vi "ShooterMech v2.vi"() -> ()   [LabVIEW 2015]
uses:
  <vilib>/Rock Robotics/WPI/Solenoid/WPI_SolenoidValue.ctl
  <vilib>/Rock Robotics/WPI/Solenoid/WPI_SolenoidSetEnum.vi
  Velocity Variable.vi
panel:
  out "Shtr":dbl
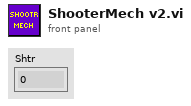
[diagram p1: front panel]
types:
  T1 = typedef "WPI_SolenoidValue.ctl" = enum16{"Off", "On", "Forward", "Reverse"}
  T2 = typedef "WPI_JoystickDevRef.ctl" = cluster{"Device":T3}
  T3 = typedef "WPI_JoystickDeviceEnum.ctl" = enum16{"USB 0", "USB 1", "USB 2", "USB 3", "USB 4", "USB 5"}
  T4 = cluster{"Buttons[0]":bool, "Buttons[1]":bool, "Buttons[2]":bool, "Buttons[3]":bool, "Buttons[4]":bool, "Buttons[5]":bool, "Buttons[6]":bool, "Buttons[7]":bool, "Buttons[8]":bool}
  T5 = typedef "WPI_SolenoidDevRef.ctl" = cluster{"DevStatus":errorcluster, "Pneumatics Control Module":u8, "Forward Solenoid Channel":T6, "Reverse Solenoid Channel":T6}
  T6 = typedef "WPI_SolenoidChannel.ctl" = enum8{"Solenoid 0", "Solenoid 1", "Solenoid 2", "Solenoid 3", "Solenoid 4", "Solenoid 5", "Solenoid 6", "Solenoid 7", "Invalid"}
  T7 = typedef "WPI_MotorControlDeviceRef.ctl" = cluster{"DeviceStatus":errorcluster, "Type":T8, "PWM":cluster{"PWM Channel":T9, "DeadBand":T10}, "CAN":cluster{"Device Number":u8, "Control Mode":T11, "Semaphore":T12, "Max Vout":dbl, "TalonSRX Control Mode":T13}, "Invert":bool}
  T8 = typedef "WPI_MotorControlType.ctl" = enum16{"PWM", "CAN", "CANTalonSRX"}
  T9 = typedef "FPGA_DIOPWMChannel.ctl" = enum8{"PWM 0", "PWM 1", "PWM 2", "PWM 3", "PWM 4", "PWM 5", "PWM 6", "PWM 7", "PWM 8", "PWM 9", "PWM MXP 0", "PWM MXP 1", "PWM MXP 2", "PWM MXP 3", "PWM MXP 4", "PWM MXP 5", "PWM MXP 6", "PWM MXP 7", "PWM MXP 8", "PWM MXP 9", "Invalid"}
  T10 = typedef "WPI_PWMDeadband.ctl" = cluster{"Name":string, "maxPositivePwm":i32, "minPositivePwm":i32, "centerPwm":i32, "maxNegativePwm":i32, "minNegativePwm":i32, "angularRange":u16}
  T11 = typedef "WPI_CANJaguar_ControlMode.ctl" = enum8{"Percent VBus", "Current", "Speed", "Position", "Voltage"}
  T12 = typedef "Semaphore RefNum" = refnum<k1>
  T13 = typedef "WPI_CANTalonSRX_APIControlMode.ctl" = enum8{"Percent VBus", "Speed", "Position", "Slave", "Unchanged / Invalid", "Voltage Compensation", "Current", "Motion Profile"}
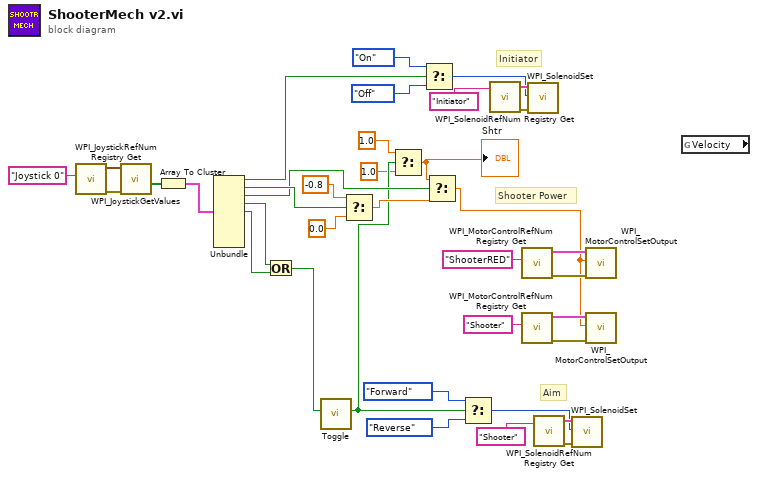
[diagram p0: block diagram]
diagram:
  # "Shooter Power"
  # "Aim"
  # "Initiator"
  n1 = call <vilib>:"WPI_JoystickRefNum Registry Get.vi"("refnum name"="Joystick 0") -> ("error out"=w25:errorcluster, "JoystickDevRef"=w24:T2)  [unwired: 9 in]
  n2 = call <vilib>:"WPI_JoystickGetValues.vi"("error in (no error)"=w25, "JoystickDevRef"=w24) -> ("Buttons"=w23:bool[])  [unwired: 5 in, 4 out]
  n3 = Array To Cluster(array=w23) -> (cluster=w22:T4)
  n4 = Unbundle(w22) -> ("Buttons[0]"=w10:bool, "Buttons[1]"=w9:bool, "Buttons[2]"=w8:bool, "Buttons[3]"=w6:bool, "Buttons[4]"=w7:bool)  [unwired: 4 out]
  n5 = Or(x=w6, y=w7) -> (x .or. y?=w5:bool)
  n6 = call "Toggle.vi"("Input"=w5) -> ("Output"=w3:bool)  [unwired: 10 in]
  n7 = Select(t=-0.8, s=w9, f=0.0) -> (s? t:f=w14:dbl)
  n8 = Select(t=1.0 ("Output"), s=w3, f=1.0) -> (s? t:f=w2:dbl)
  "Shtr" <- w2
  n9 = Select(t=WPI_SolenoidValue."On" ("Value"), s=w10, f=WPI_SolenoidValue."Off" ("Value")) -> (s? t:f=w27:T1)
  n10 = Select(t=w2, s=w8, f=w14) -> (s? t:f=w11:dbl)
  n11 = Select(t=WPI_SolenoidValue."Forward" ("Value"), s=w3, f=WPI_SolenoidValue."Reverse" ("Value")) -> (s? t:f=w17:T1)
  n12 = call <vilib>:"WPI_SolenoidRefNum Registry Get.vi"("refnum name"="Initiator") -> ("error out"=w30:errorcluster, "SolenoidDevRef"=w31:T5)  [unwired: 9 in]
  n13 = call <vilib>:"WPI_MotorControlRefNum Registry Get.vi"("refnum name"="ShooterRED") -> ("error out"=w35:errorcluster, "MotorControlDevRef"=w34:T7)  [unwired: 9 in]
  n14 = call <vilib>:"WPI_MotorControlRefNum Registry Get.vi"("refnum name"="Shooter") -> ("error out"=w33:errorcluster, "MotorControlDevRef"=w32:T7)  [unwired: 9 in]
  n15 = call-poly <vilib>:"WPI_SolenoidSet.vi"("error in (no error)"=w30, "Value"=w27, "SolenoidDevRef"=w31) -> ()  [unwired: 7 in, 2 out]
  n16 = call <vilib>:"WPI_SolenoidRefNum Registry Get.vi"("refnum name"="Shooter") -> ("error out"=w20:errorcluster, "SolenoidDevRef"=w21:T5)  [unwired: 9 in]
  n17 = call-poly <vilib>:"WPI_SolenoidSet.vi"("error in (no error)"=w20, "Value"=w17, "SolenoidDevRef"=w21) -> ()  [unwired: 7 in, 2 out]
  n18 = call <vilib>:"WPI_MotorControlSetOutput.vi"("error in (no error)"=w35, "Output"=w11, "MotorControlDevRef"=w34) -> ()  [unwired: 6 in, 3 out]
  n19 = call <vilib>:"WPI_MotorControlSetOutput.vi"("error in (no error)"=w33, "Output"=w11, "MotorControlDevRef"=w32) -> ()  [unwired: 6 in, 3 out]
  n20 = global read "Velocity Variable.vi" "Velocity"() -> ()  [unwired: 1 out]
